vi "ConvertStringBufferToArray.vi"(11 "Input String Buffer":string) -> (3 "Output Array":dbl[](array[numeric]))   [LabVIEW 2020]
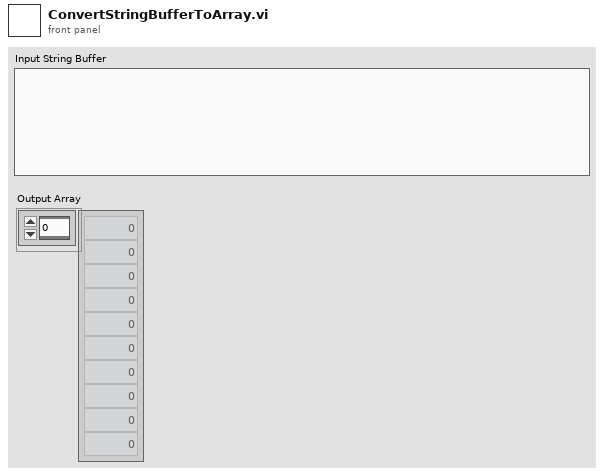
[diagram p1: front panel]
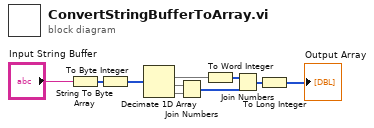
[diagram p0: block diagram]
diagram:
  n1 = String To Byte Array(string="Input String Buffer") -> (unsigned byte array=w8:u8[])
  n2 = To Byte Integer(number=w8) -> (8bit integer=w9:i8[])
  n3 = Decimate 1D Array(w9) -> (w5:i8[], w4:i8[], w3:i8[])  [unwired: 1 out]
  n4 = Join Numbers(hi=w4, lo=w3) -> ((hi.lo)=w2:u16[])
  n5 = To Word Integer(number=w5) -> (16bit integer=w6:i16[])
  n6 = Join Numbers(hi=w6, lo=w2) -> ((hi.lo)=w7:u32[])
  n7 = To Long Integer(number=w7) -> (32bit integer=→"Output Array":i32[])
